vi "Set View VI Reference.vi"(8 "error in (no error)":errorcluster, 10 "View VI Reference":refnum<vi>, 11 "View In":refnum<class "View.lvclass">) -> (0 "error out":errorcluster, 3 "View Out":refnum<class "View.lvclass">)   [LabVIEW 2020, in "View.lvclass"]
doc: "Set the reference to the View.vi. This method should be called when the View.vi is started."
uses:
  View.lvclass
  View.lvclass/View.ctl
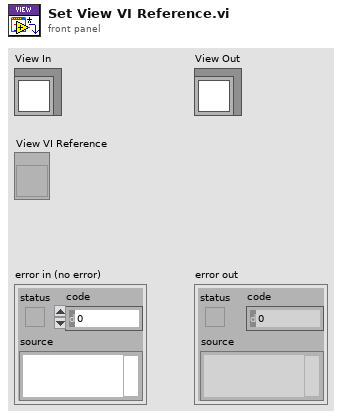
[diagram p1: front panel]
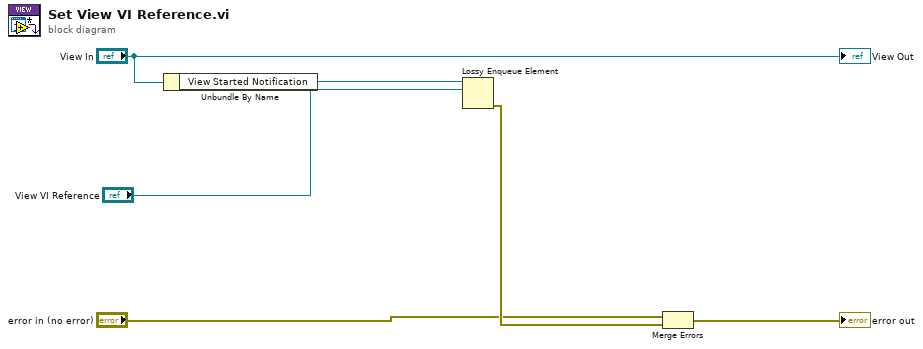
[diagram p0: block diagram]
diagram:
  n1 = Unbundle By Name("View In") -> ("View Started Notification"=w5:refnum<queue>)
  n2 = Lossy Enqueue Element(queue=w5, element="View VI Reference") -> (error out=w4:errorcluster)  [unwired: 1 in, 3 out]
  n3 = Merge Errors("error in (no error)", w4) -> (→"error out":errorcluster)
  "View Out" <- "View In"
